vi "Set Plot Type.vi"(8 "error in (no error)":errorcluster, 10 "Plot type":u16(ring) items=["X-Y Plot", "Waveform Plot"], 11 "XY WFRM Plot in":refnum<class "XY WFRM Plot.lvclass">) -> (0 "error out":errorcluster, 3 "XY WFRM Plot out":refnum<class "XY WFRM Plot.lvclass">)   [LabVIEW 2015, in "XY WFRM Plot.lvclass"]
uses:
  XY WFRM Plot.lvclass
  XY WFRM Plot.lvclass/XY WFRM Plot.ctl
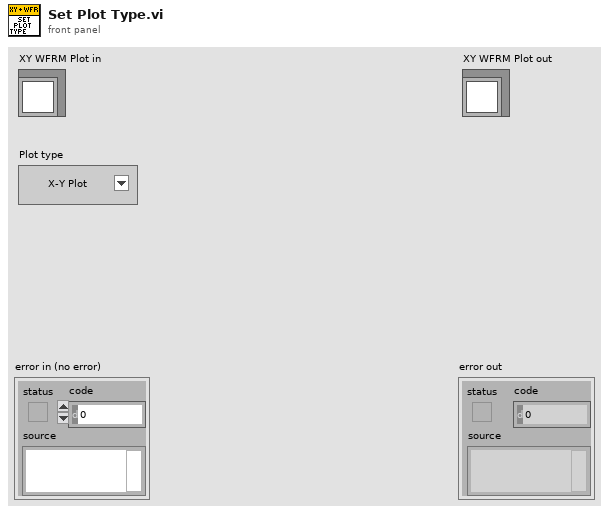
[diagram p1: front panel]
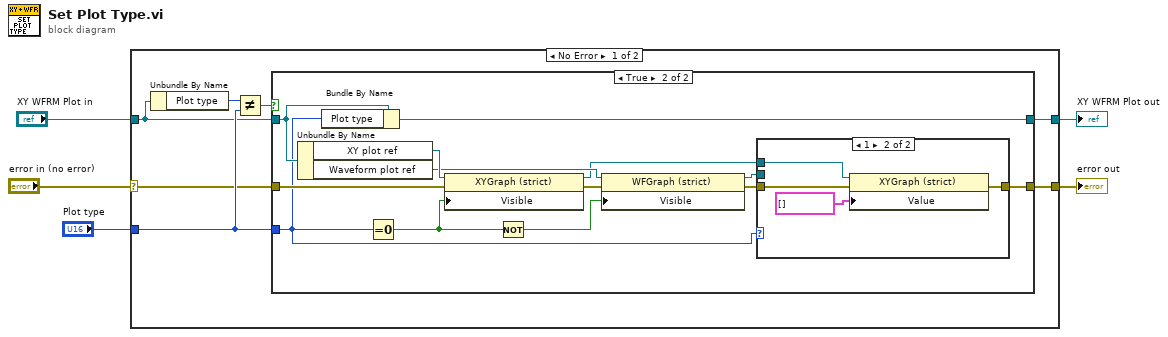
[diagram p0: block diagram]
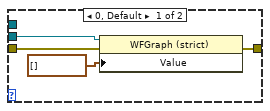
[diagram p3: hidden frame]
diagram:
  n1 = case shown="No Error" "error in (no error)" {
    selector: "error in (no error)" -> [w9 w37]
    tunnel: [w8 w37] -> w4
    tunnel: [w6 w36] -> w2
    tunnel: "XY WFRM Plot in" -> [w7 w36]
    tunnel: "Plot type" -> [w10 _]
    frame No Error {
      n2 = Unbundle By Name(w7) -> ("Plot type"=w12:u16)
      n3 = Not Equal?(x=w12, y=w10) -> (x != y?=w11:bool)
      n4 = case shown="True" w11 {
        tunnel: w10 -> [_ w16]
        tunnel: w7 -> [w14 w27]
        tunnel: w9 -> [w13 w25]
        tunnel: [w13 w17] -> w8
        tunnel: [w14 w20] -> w6
        frame False {
        }
        frame True {
          n5 = Unbundle By Name(w27) -> ("XY plot ref"=w26:refnum<vi>, "Waveform plot ref"=w24:refnum<vi>)
          n6 = Bundle By Name(cluster=w27, "Plot type"=w16) -> (w20:refnum<class "XY WFRM Plot.lvclass">)
          n7 = Equal To 0?(x=w16) -> (x = 0?=w23:bool)
          n8 = property class="XYGraph (strict)"(reference=w26, error in=w25, "Visible"=w23) -> (reference out=w15:refnum<vi>, error out=w21:errorcluster)
          n9 = Not(x=w23) -> (.not. x?=w22:bool)
          n10 = property class="WFGraph (strict)"(reference=w24, error in=w21, "Visible"=w22) -> (reference out=w18:refnum<vi>, error out=w19:errorcluster)
          n11 = case shown="1" w16 {
            tunnel: w19 -> [w31 w35]
            tunnel: w18 -> [w30 _]
            tunnel: [w29 w34] -> w17
            tunnel: w15 -> [_ w33]
            frame 0, Default {
              n12 = property class="WFGraph (strict)"(reference=w30, error in=w31, "Value"=waveform(sgl)[] []) -> (error out=w29:errorcluster)  [unwired: 1 out]
            }
            frame 1 {
              n13 = property class="XYGraph (strict)"(reference=w33, error in=w35, "Value"=cluster{"Y":sgl[], "Y":sgl[]}[] []) -> (error out=w34:errorcluster)  [unwired: 1 out]
            }
          }
        }
      }
    }
    frame Error {
    }
  }
  "error out" <- w4
  "XY WFRM Plot out" <- w2
